vi "SetClusterValue-rec.vi"(0 "VI Reference":refnum<vi>, 5 "Array":string[](array[string]), 7 "Control Value":variant, 11 "error in":errorcluster) -> (4 "VI Reference out":refnum<vi>, 15 "error out":errorcluster)   [LabVIEW 2016]
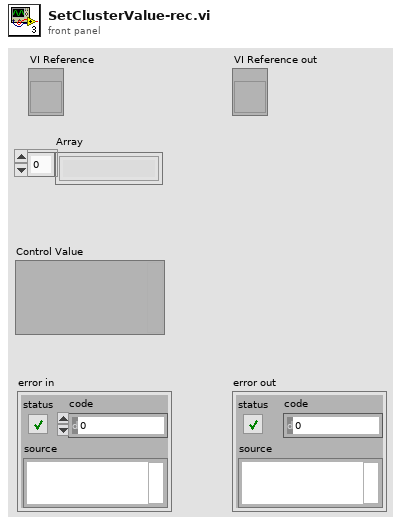
[diagram p1: front panel]
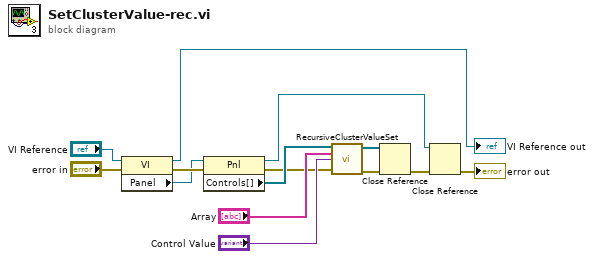
[diagram p0: block diagram]
diagram:
  n1 = property class="VI"(reference="VI Reference", error in="error in") -> (reference out=→"VI Reference out":refnum<vi>, error out=w14:errorcluster, "Panel"=w13:refnum<vi>)
  n2 = property class="Pnl"(reference=w13, error in=w14) -> (reference out=w9:refnum<vi>, error out=w4:errorcluster, "Controls[]"=w7:refnum<vi>[])
  n3 = call "RecursiveClusterValueSet.vi"("Controls[] In"=w7, "Array"="Array", "Control Value"="Control Value", "error in (no error)"=w4) -> ("Controls[] Out"=w1:refnum<vi>[], "error out"=w3:errorcluster)  [unwired: 10 in]
  n4 = Close Reference(reference=w1, error in (no error)=w3) -> (error out=w2:errorcluster)
  n5 = Close Reference(reference=w9, error in (no error)=w2) -> (error out=→"error out":errorcluster)
